vi "int_to_LV_time.vi"(7 "error in (no error)":errorcluster, 10 "Integer Timestamp":i64) -> (0 "error out":errorcluster, 3 "time stamp":timestamp)   [LabVIEW 2013]
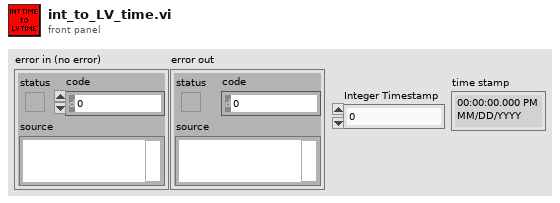
[diagram p1: front panel]
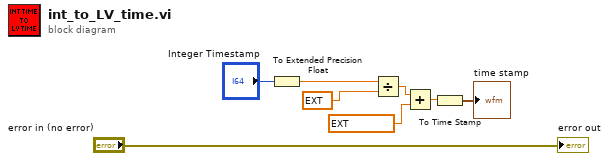
[diagram p0: block diagram]
diagram:
  n1 = To Extended Precision Float(1:"Integer Timestamp") -> (0:w3:ext)
  n2 = Divide(x=w3, y=ext 1000.0) -> (x/y=w2:ext)
  n3 = Add(x=w2, y=ext 2082844800.0) -> (x+y=w1:ext)
  n4 = To Time Stamp(1:w1) -> (0:→"time stamp":timestamp)
  "error out" <- "error in (no error)"
